vi "Stop Executions.vi"(8 "error in (no error)":errorcluster, 10 "Main Continer":refnum<vi>, 11 "Application in":refnum<data-value>) -> (0 "error out":errorcluster, 3 "Application out":refnum<data-value>)   [LabVIEW 2015, in "Application.lvclass"]
uses:
  Application.lvclass
  Execution.lvclass
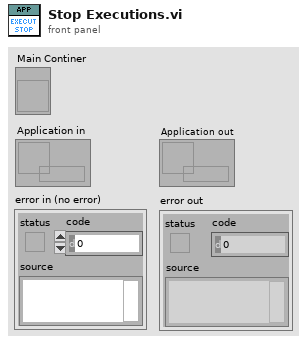
[diagram p1: front panel]
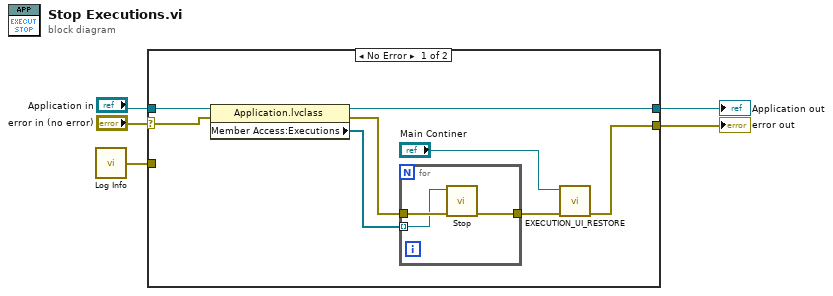
[diagram p0: block diagram]
diagram:
  n1 = call "Log Info.vi"() -> ("error out"=w3:errorcluster)  [unwired: 5 in]
  n2 = case shown="No Error" "error in (no error)" {
    selector: "error in (no error)" -> [w10 w17]
    tunnel: [w8 w17] -> w4
    tunnel: [w12 w16] -> w1
    tunnel: "Application in" -> [w12 w16]
    tunnel: w3 -> [_ _]
    frame No Error {
      n3 = property class="Application.lvclass"(reference=w12, error in=w10) -> (error out=w9:errorcluster, "Member Access:Executions"=w11:refnum<data-value>[])  [unwired: 1 out]
      n4 = for {
        tunnel: w11 -> [w14] mode=indexing
        tunnel: w9 -> [w15]
        tunnel: [w13] -> w6
        n5 = call "Stop.vi"("error in (no error)"=w15, "Execution in"=w14) -> ("error out"=w13:errorcluster)  [unwired: 8 in, 1 out]
      }
      n6 = call "EXECUTION_UI_RESTORE.vi"("error in (no error)"=w6, "Main Continer"="Main Continer") -> ("error out"=w8:errorcluster)  [unwired: 9 in]
    }
    frame Error {
    }
  }
  "error out" <- w4
  "Application out" <- w1
